vi "PCO_Segment.vi"() -> (0 "PCO_Segment":T1, 1 "PCO_Segment_Raw":T2, 2 "Length":u16, 3 "Raw_Length":u16)   [LabVIEW 2019, in "SDK.lvlib" / "Structures.lvlib"]
doc: "Use this template to build a VI to use as a subVI."
uses:
  Structures.lvlib
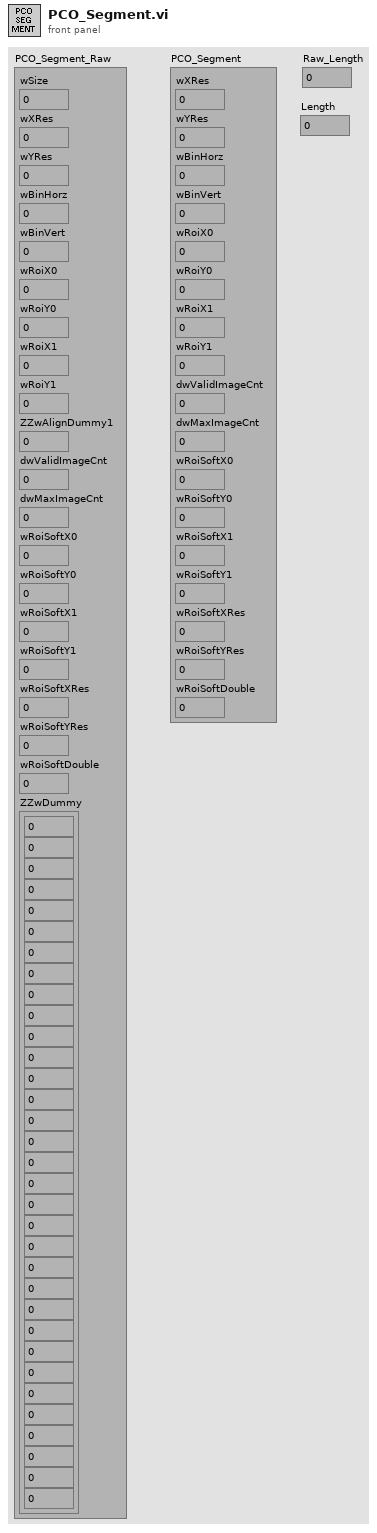
[diagram p1: front panel]
types:
  T1 = cluster{"wXRes":u16, "wYRes":u16, "wBinHorz":u16, "wBinVert":u16, "wRoiX0":u16, "wRoiY0":u16, "wRoiX1":u16, "wRoiY1":u16, "dwValidImageCnt":u32, "dwMaxImageCnt":u32, "wRoiSoftX0":u16, "wRoiSoftY0":u16, "wRoiSoftX1":u16, "wRoiSoftY1":u16, "wRoiSoftXRes":u16, "wRoiSoftYRes":u16, "wRoiSoftDouble":u16}
  T2 = cluster{"wSize":u16, "wXRes":u16, "wYRes":u16, "wBinHorz":u16, "wBinVert":u16, "wRoiX0":u16, "wRoiY0":u16, "wRoiX1":u16, "wRoiY1":u16, "ZZwAlignDummy1":u16, "dwValidImageCnt":u32, "dwMaxImageCnt":u32, "wRoiSoftX0":u16, "wRoiSoftY0":u16, "wRoiSoftX1":u16, "wRoiSoftY1":u16, "wRoiSoftXRes":u16, "wRoiSoftYRes":u16, "wRoiSoftDouble":u16, "ZZwDummy":cluster{u16, u16, u16, u16, u16, u16, u16, u16, u16, u16, u16, u16, u16, u16, u16, u16, u16, u16, u16, u16, u16, u16, u16, u16, u16, u16, u16, u16, u16, u16, u16, u16, u16}}
  T3 = cluster{u16, u16, u16, u16, u16, u16, u16, u16, u16, u16, u16, u16, u16, u16, u16, u16, u16, u16, u16, u16, u16, u16, u16, u16, u16, u16, u16, u16, u16, u16, u16, u16, u16}
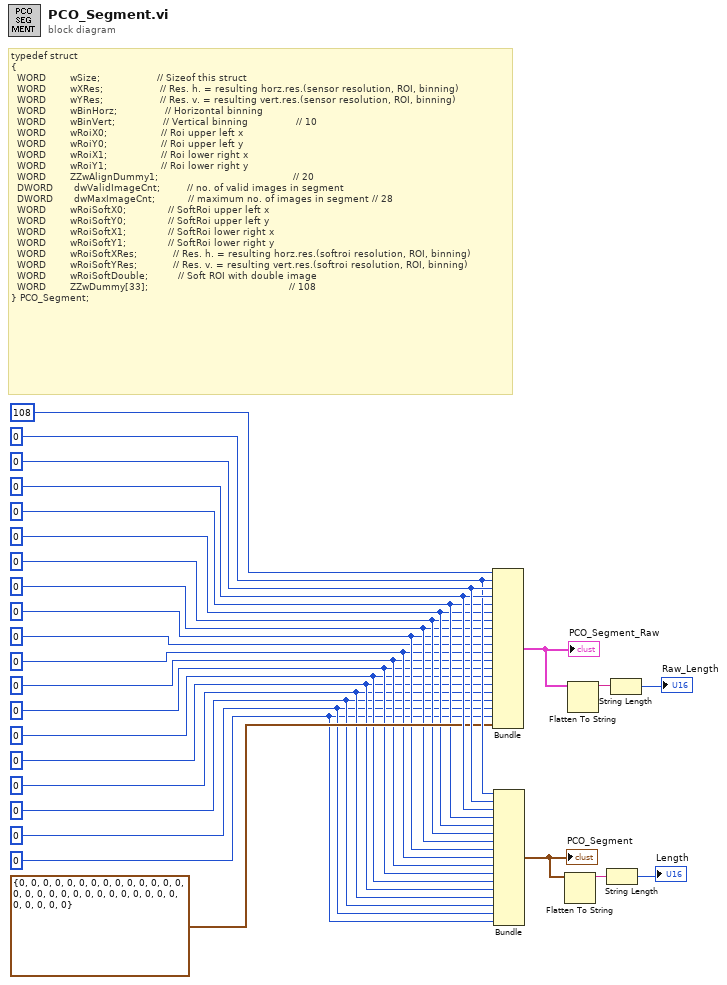
[diagram p0: block diagram]
diagram:
  w1 = u16 0 ("wRoiSoftDouble")
  w3 = u16 0 ("wRoiSoftYRes")
  w4 = u16 0 ("wRoiSoftXRes")
  w5 = u16 0 ("wRoiSoftY1")
  w6 = u16 0 ("wRoiSoftX1")
  w7 = u16 0 ("wRoiSoftY0")
  w8 = u16 0 ("wRoiSoftX0")
  w9 = u32 0 ("dwMaxImageCnt")
  w10 = u32 0 ("dwValidImageCnt")
  w12 = u16 0 ("wRoiY1")
  w13 = u16 0 ("wRoiX1")
  w14 = u16 0 ("wRoiY0")
  w15 = u16 0 ("wRoiX0")
  w16 = u16 0 ("wBinVert")
  w19 = u16 0 ("wBinHorz")
  w20 = u16 0 ("wYRes")
  w18 = u16 0 ("wXRes")
  # "typedef struct\n{\n  WORD        wSize;                   // Sizeof this struct\n  WORD        wXRes;                   // Res. h. = resulting horz.res.(sensor resolution, ROI, binning)\n  WORD        wYRes;                   // Res. v. = resulting vert.res.(sensor resolution, ROI, binning)\n  WORD        wBinHorz;                // Horizontal binning\n  WORD        wBinVert;                // Vertical binning                // 10\n  WORD        wRoiX0;                  // Roi upper left x\n  WORD        wRoiY0;                  // Roi upper left y\n  WORD        wRoiX1;                  // Roi lower right x\n  WORD        wRoiY1;                  // Roi lower right y\n  WORD        ZZwAlignDummy1;                                             // 20\n  DWORD       dwValidImageCnt;         // no. of valid images in segment\n  DWORD       dwMaxImageCnt;           // maximum no. of images in segment // 28\n  WORD        wRoiSoftX0;              // SoftRoi upper left x\n  WORD        wRoiSoftY0;              // SoftRoi upper left y\n  WORD        wRoiSoftX1;              // SoftRoi lower right x\n  WORD        wRoiSoftY1;              // SoftRoi lower right y\n  WORD        wRoiSoftXRes;            // Res. h. = resulting horz.res.(softroi resolution, ROI, binning)\n  WORD        wRoiSoftYRes;            // Res. v. = resulting vert.res.(softroi resolution, ROI, binning)\n  WORD        wRoiSoftDouble;          // Soft ROI with double image\n  WORD        ZZwDummy[33];                                               // 108\n} PCO_Segment;"
  n1 = Bundle("wSize"=u16 108, "wXRes"=w18, "wYRes"=w20, "wBinHorz"=w19, "wBinVert"=w16, "wRoiX0"=w15, "wRoiY0"=w14, "wRoiX1"=w13, "wRoiY1"=w12, "ZZwAlignDummy1"=u16 0, "dwValidImageCnt"=w10, "dwMaxImageCnt"=w9, "wRoiSoftX0"=w8, "wRoiSoftY0"=w7, "wRoiSoftX1"=w6, "wRoiSoftY1"=w5, "wRoiSoftXRes"=w4, "wRoiSoftYRes"=w3, "wRoiSoftDouble"=w1, "ZZwDummy"=T3 {0, 0, 0, 0, 0, 0, 0, 0, 0, 0, 0, 0, 0, 0, 0, 0, 0, 0, 0, 0, 0, 0, 0, 0, 0, 0, 0, 0, 0, 0, 0, 0, 0}) -> (w21:T2)  [unwired: 1 in]
  "PCO_Segment_Raw" <- w21
  n2 = Bundle("wXRes"=w18, "wYRes"=w20, "wBinHorz"=w19, "wBinVert"=w16, "wRoiX0"=w15, "wRoiY0"=w14, "wRoiX1"=w13, "wRoiY1"=w12, "dwValidImageCnt"=w10, "dwMaxImageCnt"=w9, "wRoiSoftX0"=w8, "wRoiSoftY0"=w7, "wRoiSoftX1"=w6, "wRoiSoftY1"=w5, "wRoiSoftXRes"=w4, "wRoiSoftYRes"=w3, "wRoiSoftDouble"=w1) -> (w2:T1)  [unwired: 1 in]
  "PCO_Segment" <- w2
  n3 = Flatten To String(anything=w2) -> (data string=w26:string)  [unwired: 3 in, 2 out]
  n4 = Flatten To String(anything=w21) -> (data string=w25:string)  [unwired: 3 in, 2 out]
  n5 = String Length(string=w26) -> (length=→"Length":i32)
  n6 = String Length(string=w25) -> (length=→"Raw_Length":i32)
